vi "Addup.vi"(3 "error in (no error)":errorcluster, 4 "Length":i32, 5 "queue in":refnum<queue>) -> (0 "error out":errorcluster, 1 "Byte Array":u8[](array[numeric]), 2 "queue out":refnum<queue>)   [LabVIEW 2014]
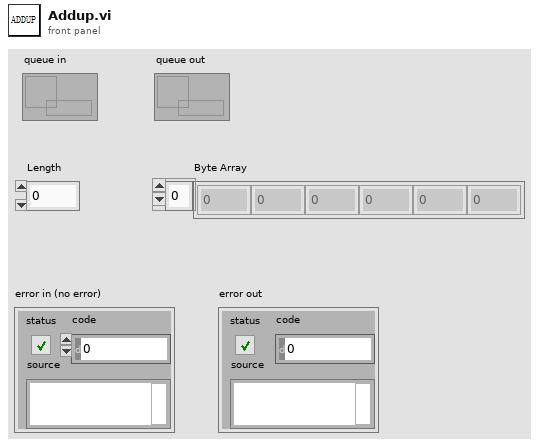
[diagram p1: front panel]
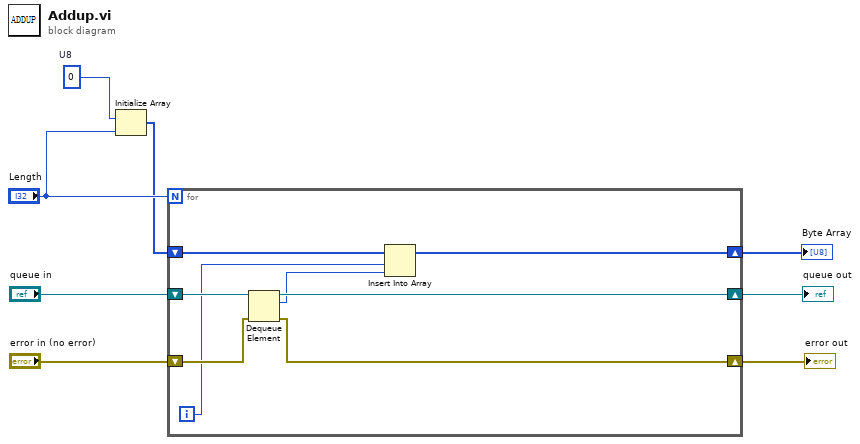
[diagram p0: block diagram]
diagram:
  w6 = u8 0  # U8
  n1 = Initialize Array(w6, "Length") -> (w4:u8[])
  n2 = for {
    N: "Length" -> [_]
    shift-right: [w14] -> w7
    shift-left: "error in (no error)" -> [w15]
    shift-right: [w13] -> w1
    shift-left: "queue in" -> [w16]
    shift-right: [w11] -> w3
    shift-left: w4 -> [w12]
    i -> [w10]
    n3 = Dequeue Element(queue=w16, error in (no error)=w15) -> (queue out=w13:refnum<queue>, element=w9:u8, error out=w14:errorcluster)  [unwired: 1 in, 1 out]
    n4 = Insert Into Array(array=w12, index=w10, new element=w9) -> (w11:u8[])
  }
  "error out" <- w7
  "Byte Array" <- w3
  "queue out" <- w1
